vi "Read (In Place).vi"(8 "error in (no error)":errorcluster, 9 "timeout us (-1)":i64=-1, 10 "preallocated data in":string, 11 "pipe reader in":refnum<data-value>) -> (0 "error out":errorcluster, 1 "bytes read":i32, 2 "data out":string, 3 "pipe reader out":refnum<data-value>, 4 "timed out?":bool)   [LabVIEW 2013, in "Linux RT IPC.Pipes.lvlib" / "Unix Pipe Reader.lvclass"]
doc: "This VI reads a certain number of bytes from the provided pipe endpoint."
uses:
  Unix Pipe Reader.lvclass
  Unix Pipe Reader.lvclass/Unix Pipe Reader.ctl
  Unix Pipe/Unix Pipe.lvclass/Unix Pipe.ctl
  <vilib>/NI/NI Linux RT Utilities/VIs/Public/Convert Types/convert timespec 64 to timespec 32.vi
  <vilib>/NI/NI Linux RT Utilities/VIs/Public/Convert Types/convert timespec 32 to timespec 64.vi
  C/SubVIs/error handler.vi
  <vilib>/NI/NI Linux RT Errno/VIs/Public/Get Errno Value for Calling Thread.vi
  <vilib>/NI/NI Linux RT Errno/VIs/Public/SubVIs/get errno from error code.vi
  Unix Pipe/Unix Pipe.lvclass
  C/Linux RT IPC.C.lvlib
  <vilib>/NI/NI Linux RT Utilities/Linux RT Utilities.lvlib
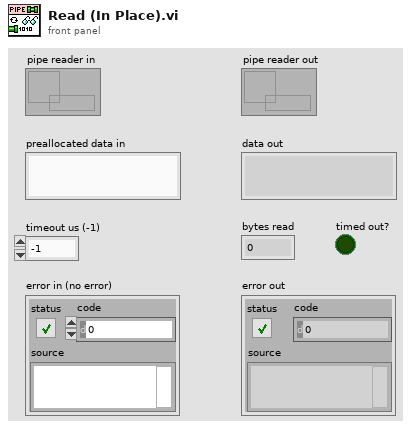
[diagram p1: front panel]
types:
  T1 = cluster{"it_interval":cluster{"sec":u64, "nsec":u64}, "it_value":cluster{"sec":u64, "nsec":u64}}
  T2 = typedef "Linux RT IPC.C.lvlib/epoll event struct.ctl" = cluster{"events":u32, "data":u64}
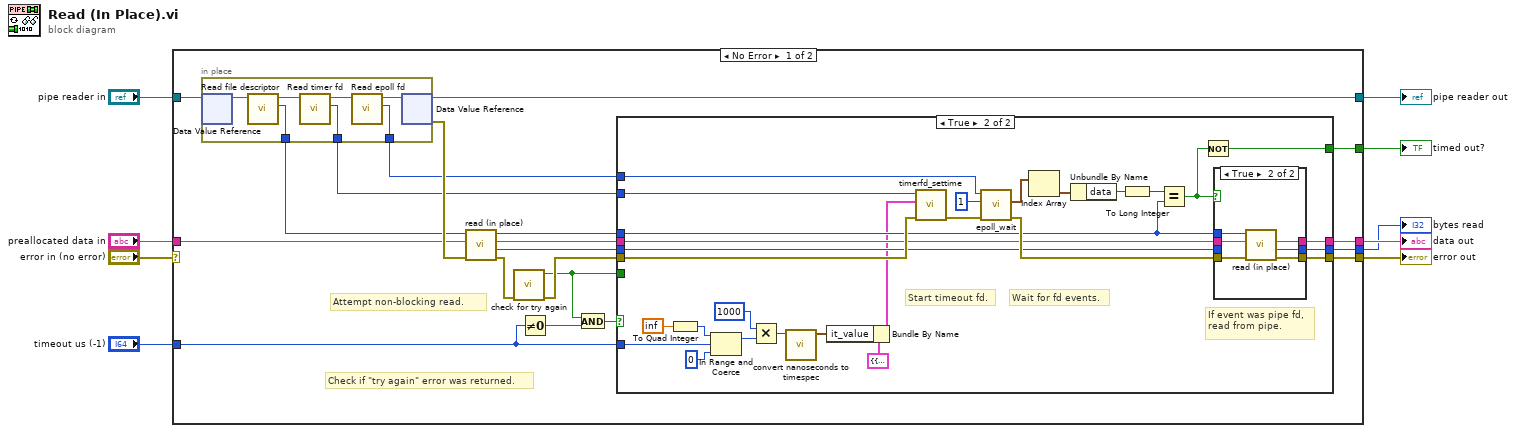
[diagram p0: block diagram]
diagram:
  n1 = case shown="No Error" "error in (no error)" {
    selector: "error in (no error)" -> [_ w79]
    tunnel: "pipe reader in" -> [w28 w80]
    tunnel: [w10 w80] -> w7
    tunnel: [w24 w79] -> w6
    tunnel: [w23 _] -> w1
    tunnel: [w22 w78] -> w5
    tunnel: "timeout us (-1)" -> [w14 _]
    tunnel: [w19 _] -> w3
    tunnel: "preallocated data in" -> [w13 w78]
    frame No Error {
      # "Check if \"try again\" error was returned."
      # "Attempt non-blocking read."
      n2 = in-place {
        in-place-border: [w77] -> w27
        in-place-border: [w76] -> w12
        in-place-border: [w75] -> w11
        n3 = in-place-dvr #1(w28) -> (w74:refnum<class "Unix Pipe Reader.lvclass">)  [unwired: 1 out]
        n4 = call "Read file descriptor.vi"("Unix Pipe in"=w74) -> ("file descriptor"=w77:i32, "Unix Pipe out"=w73:refnum<class "Unix Pipe Reader.lvclass">)  [unwired: 8 in, 1 out]
        n5 = call "Read timer fd.vi"("Unix Pipe Reader in"=w73) -> ("timer fd"=w76:i32, "Unix Pipe Reader out"=w72:refnum<class "Unix Pipe Reader.lvclass">)  [unwired: 8 in, 1 out]
        n6 = call "Read epoll fd.vi"("Unix Pipe Reader in"=w72) -> ("epoll fd"=w75:i32, "Unix Pipe Reader out"=w71:refnum<class "Unix Pipe Reader.lvclass">)  [unwired: 8 in, 1 out]
        n7 = in-place-dvr #1(w71) -> (w10:refnum<data-value>, w29:errorcluster)
      }
      n8 = call "read (in place).vi"("error in (no error)"=w29, "preallocated data in"=w13, "file descriptor in"=w27) -> ("error out"=w21:errorcluster, "bytes read"=w25:i32, "data out"=w15:string, "file descriptor out"=w26:i32)  [unwired: 5 in]
      n9 = call "check for try again.vi"("error in (no error)"=w21) -> ("error out"=w18:errorcluster, "try again?"=w17:bool)  [unwired: 9 in]
      n10 = Not Equal To 0?(x=w14) -> (x != 0?=w16:bool)
      n11 = And(x=w17, y=w16) -> (x .and. y?=w20:bool)
      n12 = case shown="True" w20 {
        tunnel: w26 -> [_ w44]
        tunnel: w15 -> [w31 w39]
        tunnel: w25 -> [w32 w38]
        tunnel: w18 -> [w33 w61]
        tunnel: [w33 w49] -> w24
        tunnel: [w32 w46] -> w23
        tunnel: [w31 w50] -> w22
        tunnel: w14 -> [_ w56]
        tunnel: [w30 w47] -> w19
        tunnel: w17 -> [w30 _]
        tunnel: w12 -> [_ w36]
        tunnel: w11 -> [_ w35]
        frame False {
          # "Either try again was false (pipe read was successfully), another error occurred, or the user specified a timeout of zero, so no retry should be made."
        }
        frame True {
          # "If event was pipe fd, read from pipe."
          # "Wait for fd events."
          # "Start timeout fd."
          n13 = To Quad Integer(1:inf) -> (0:w40:i64)
          n14 = In Range and Coerce(upper limit=w40, x=w56, lower limit=i64 0) -> (coerced(x)=w43:i64)  [unwired: 1 out]
          n15 = Multiply(x=i64 1000, y=w43) -> (x*y=w42:i64)
          n16 = call <vilib>:"convert nanoseconds to timespec.vi"("nanoseconds"=w42) -> ("timespec"=w57:cluster{"sec":u64, "nsec":u64})  [unwired: 10 in]
          n17 = Bundle By Name(cluster=T1 {"it_interval"={"sec"=0, "nsec"=0}, "it_value"={"sec"=0, "nsec"=0}} ("new value"), "it_value"=w57) -> (w34:T1)
          n18 = call "timerfd_settime.vi"("error in (no error)"=w61, "new value"=w34, "fd in"=w36) -> ("error out"=w48:errorcluster)  [unwired: 6 in, 2 out]
          n19 = call "epoll_wait.vi"("error in (no error)"=w48, "max events"=u32 1, "epfd in"=w35) -> ("error out"=w55:errorcluster, "events"=w52:T2[])  [unwired: 4 in, 3 out]
          n20 = Index Array(array=w52) -> (element=w53:T2)  [unwired: 1 in]
          n21 = Unbundle By Name(w53) -> ("data"=w54:u64)
          n22 = To Long Integer(number=w54) -> (32bit integer=w45:i32)
          n23 = Equal?(x=w45, y=w44) -> (x = y?=w37:bool)
          n24 = Not(x=w37) -> (.not. x?=w47:bool)
          n25 = case shown="True" w37 {
            tunnel: [w63 w70] -> w50
            tunnel: [w62 w69] -> w46
            tunnel: [w64 w68] -> w49
            tunnel: w55 -> [w64 w67]
            tunnel: w44 -> [_ w66]
            tunnel: w39 -> [w63 w65]
            tunnel: w38 -> [w62 _]
            frame False {
            }
            frame True {
              n26 = call "read (in place).vi"("error in (no error)"=w67, "preallocated data in"=w65, "file descriptor in"=w66) -> ("error out"=w68:errorcluster, "bytes read"=w69:i32, "data out"=w70:string)  [unwired: 5 in, 1 out]
            }
          }
        }
      }
    }
    frame Error {
    }
  }
  "error out" <- w6
  "pipe reader out" <- w7
  "bytes read" <- w1
  "data out" <- w5
  "timed out?" <- w3
